vi "humidite et temperature.vi"() -> ()   [LabVIEW 2021]
uses:
  <vilib>/Utility/file.llb/Write Delimited Spreadsheet (string).vi
panel:
  out "humidite":dbl(knob) scale=0.0..100.0
  in  "stop":bool
  out "error out 4":errorcluster
  out "new file path (Not A Path if cancelled)":path
  out "error out 3":errorcluster
  out "error out 2":errorcluster
  in  "Table Control":string[][](table)
  in  "M/A":bool
  in  "clim":bool
  in  "chauff":bool
  out "ventilatteur":bool
  out "climatisuer":bool
  out "dhumidite":dbl(graph)
  out "dtemperature":dbl(graph)
  in  "VISA resource name":refnum<visa-resource-name>
  out "error out":errorcluster
  out "temperature":dbl(slide) scale=0.0..100.0
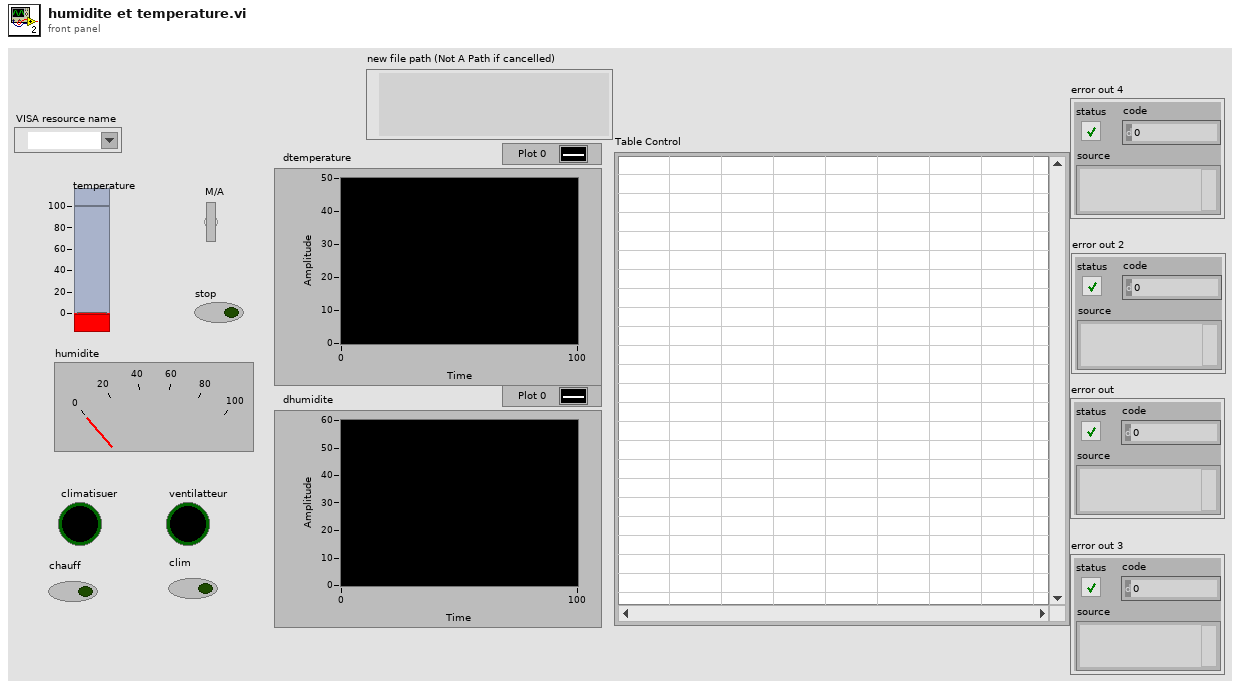
[diagram p1: front panel]
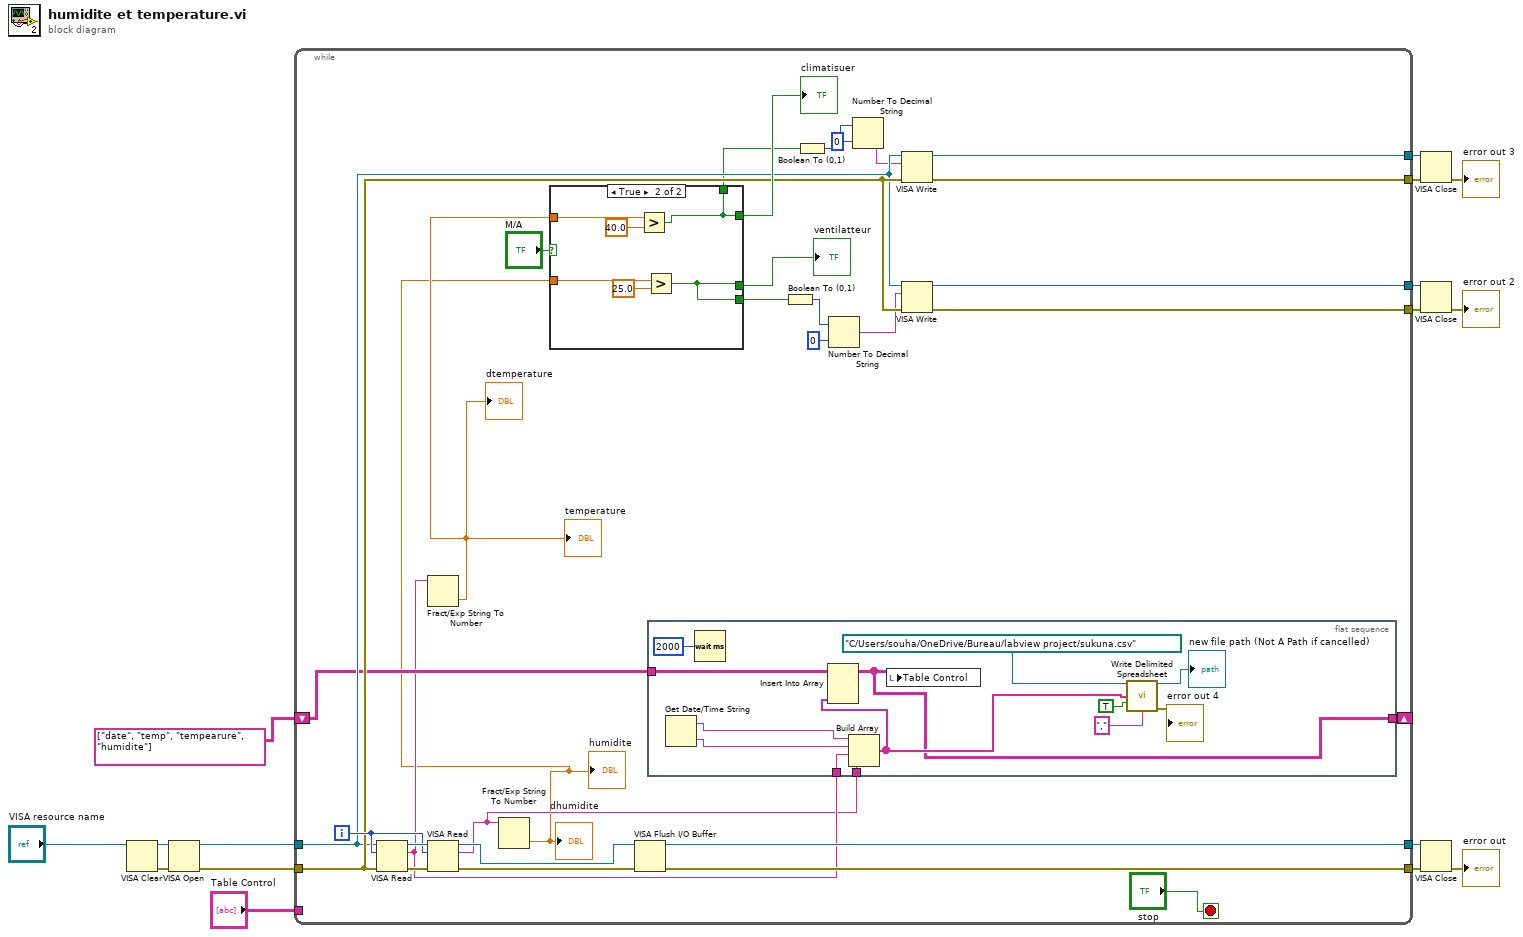
[diagram p0: block diagram]
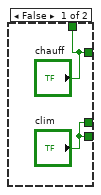
[diagram p2: hidden frame]
diagram:
  n1 = VISA Clear(VISA resource name="VISA resource name") -> (VISA resource name out=w15:refnum<visa-resource-name>, error out=w14:errorcluster)  [unwired: 1 in]
  n2 = VISA Open(error in (no error)=w14, VISA resource name=w15) -> (VISA resource name=w9:refnum<visa-resource-name>, error out=w10:errorcluster)  [unwired: 3 in]
  n3 = while {
    tunnel: [w47] -> w12
    tunnel: [w46] -> w11
    tunnel: w10 -> [w33]
    tunnel: w9 -> [w32]
    tunnel: "Table Control" -> [_]
    tunnel: [w37] -> w7
    tunnel: [w36] -> w6
    tunnel: [w35] -> w5
    tunnel: [w34] -> w4
    shift-right: [w29] -> _
    shift-left: string[][] [["date", "temp", "tempearure", "humidite"]] -> [w30]
    i -> [w41]
    stop <- "stop" stop-if-true
    n4 = VISA Read(VISA resource name=w32, byte count=w41, error in (no error)=w33) -> (VISA resource name out=w45:refnum<visa-resource-name>, read buffer=w28:string, error out=w42:errorcluster)  [unwired: 1 out]
    n5 = Fract/Exp String To Number(string=w28) -> (number=w18:dbl)  [unwired: 3 in, 1 out]
    "temperature" <- w18
    "dtemperature" <- w18
    n6 = VISA Read(VISA resource name=w45, byte count=w41, error in (no error)=w42) -> (VISA resource name out=w44:refnum<visa-resource-name>, read buffer=w19:string, error out=w43:errorcluster)  [unwired: 1 out]
    n7 = Fract/Exp String To Number(string=w19) -> (number=w17:dbl)  [unwired: 3 in, 1 out]
    "dhumidite" <- w17
    "humidite" <- w17
    n8 = case shown="True" "M/A" {
      tunnel: ["chauff" w68] -> w39
      tunnel: ["clim" w67] -> w38
      tunnel: ["chauff" w68] -> w27
      tunnel: ["clim" w67] -> w26
      tunnel: w18 -> [_ w66]
      tunnel: w17 -> [_ w65]
      frame False {
      }
      frame True {
        n9 = Greater?(x=w66, y=40.0) -> (0:w68:bool)
        n10 = Greater?(x=w65, y=25.0) -> (0:w67:bool)
      }
    }
    "climatisuer" <- w39
    "ventilatteur" <- w38
    n11 = VISA Flush I/O Buffer(VISA resource name=w44, error in (no error)=w43) -> (VISA resource name out=w47:refnum<visa-resource-name>, error out=w46:errorcluster)  [unwired: 1 in]
    n12 = flat-sequence {
      tunnel: w28 -> [w55]
      tunnel: w19 -> [w54]
      tunnel: w30 -> [w49]
      tunnel: [w48] -> w29
      frame #0 {
        n13 = Get Date/Time String() -> (date string=w52:string, time string=w51:string)  [unwired: 3 in]
        n14 = Wait (ms)(milliseconds to wait=u32 2000) -> ()  [unwired: 1 out]
        n15 = Build Array(w52, w51, w55, w54) -> (w50:string[])
        n16 = Insert Into Array(array=w49, new element=w50) -> (w48:string[][])  [unwired: 2 in]
        n17 = local write "Table Control"(w48) -> ()
        n18 = call-poly <vilib>:"Write Delimited Spreadsheet.vi"("file path (dialog if empty)"=path "C:/Users/souha/OneDrive/Bureau/labview project/sukuna.csv" ("name or relative path"), "1D data"=w50, "append to file? (new file:F)"=TRUE, "delimiter (\\t)"="," ("delimiter (\\t)")) -> ("new file path (Not A Path if cancelled)"=→"new file path (Not A Path if cancelled)":path, "error out"=→"error out 4":errorcluster)  [unwired: 10 in]
      }
    }
    n19 = Boolean To (0,1)(Boolean=w26) -> (0, 1=w22:i16)
    n20 = Boolean To (0,1)(Boolean=w27) -> (0, 1=w25:i16)
    n21 = Number To Decimal String(number=w22, width (-)=i16 0) -> (decimal integer string=w21:string)
    n22 = Number To Decimal String(number=w25, width (-)=i16 0) -> (decimal integer string=w24:string)
    n23 = VISA Write(VISA resource name=w32, write buffer=w24, error in (no error)=w33) -> (VISA resource name out=w37:refnum<visa-resource-name>, error out=w36:errorcluster)  [unwired: 1 out]
    n24 = VISA Write(VISA resource name=w32, write buffer=w21, error in (no error)=w33) -> (VISA resource name out=w35:refnum<visa-resource-name>, error out=w34:errorcluster)  [unwired: 1 out]
  }
  n25 = VISA Close(VISA resource name=w7, error in (no error)=w6) -> (error out=→"error out 3":errorcluster)
  n26 = VISA Close(VISA resource name=w5, error in (no error)=w4) -> (error out=→"error out 2":errorcluster)
  n27 = VISA Close(VISA resource name=w12, error in (no error)=w11) -> (error out=→"error out":errorcluster)
